vi "Add New Enum Node.vi"(7 "Enum Members":cluster{"Name":string, "Documentation":string}[](array[cluster]), 9 "Type Name":string, 10 "CodeDocumentation":string, 11 "Doc Ref":refnum<k20>) -> (1 "Updated Node Ref":refnum<k20>)   [LabVIEW 2025]
uses:
  <resource>/objmgr/DOMUserDefRef.rc
  Shared/Types/NodeFilteringOptions.ctl
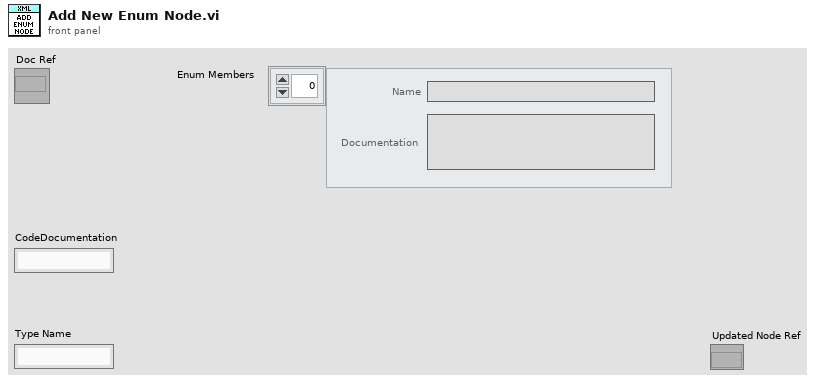
[diagram p1: front panel]
types:
  T1 = typedef "NodeFilteringOptions.ctl" = enum16{"GetCustomDeviceNode", "GetAllChannelNodes", "GetAllSectionNodes", "GetAllWaveformNodes", "GetFirstChannelNode", "GetFirstSectionNode", "GetFirstWaveformNode", "GetSpecificSectionNode", "GetSpecificCustomDeviceNode", "GetSpecificChannelNode", "GetSpecificWaveformNode", "GetMatchedNamedNode", "GetEnumDefinitionsNode", "GetSpecificEnumDefinitionNode", "GetAllEnumDefinitionNodes", "GetDynamicChannelNodes"}
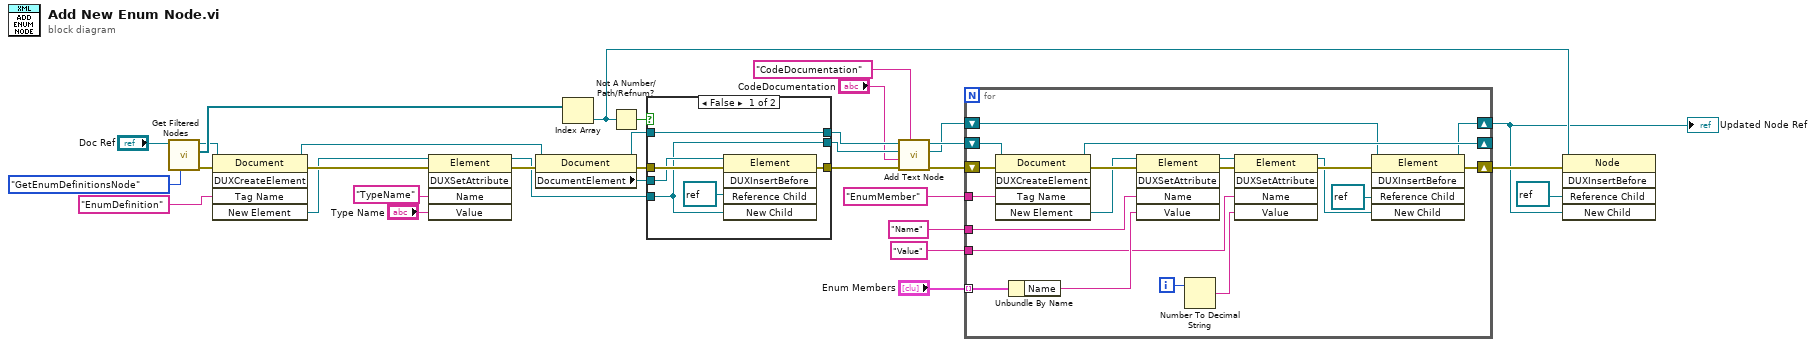
[diagram p0: block diagram]
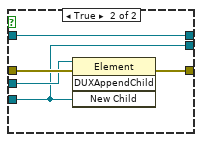
[diagram p2: hidden frame]
diagram:
  n1 = call "Get Filtered Nodes.vi"("Node Filtering"=NodeFilteringOptions."GetEnumDefinitionsNode" ("NodeFiltering"), "Document in"="Doc Ref") -> ("error out"=w22:errorcluster, "Filtered Nodes"=w21:refnum<k20>[], "Document out"=w20:refnum<k20>)  [unwired: 5 in, 2 out]
  n2 = invoke class="Document" method="DUXCreateElement"(reference=w20, error in=w22, "Tag Name"="EnumDefinition") -> (reference out=w24:refnum<k20>, error out=w33:errorcluster, "New Element"=w27:refnum<k20>)  [unwired: 2 in, 2 out]
  n3 = invoke class="Element" method="DUXSetAttribute"(reference=w27, error in=w33, "Name"="TypeName", "Value"="Type Name") -> (reference out=w26:refnum<k20>, error out=w30:errorcluster)  [unwired: 1 in, 3 out]
  n4 = property class="Document"(reference=w24, error in=w30) -> (reference out=w23:refnum<k20>, error out=w25:errorcluster, "DocumentElement"=w29:refnum<k20>)
  n5 = Index Array(array=w21) -> (element=w3:refnum<k20>)  [unwired: 1 in]
  n6 = Not A Number/Path/Refnum?(number/path/refnum=w3) -> (NaN/Path/Refnum?=w28:bool)
  n7 = case shown="False" w28 {
    tunnel: w25 -> [w39 w44]
    tunnel: [w37 w41] -> w17
    tunnel: w26 -> [w35 w40]
    tunnel: w29 -> [w38 w43]
    tunnel: w23 -> [w36 w42]
    tunnel: [w36 w42] -> w15
    tunnel: [w35 w40] -> w16
    frame False {
      n8 = invoke class="Element" method="DUXInsertBefore"(reference=w38, error in=w39, "Reference Child"=refnum<k20> refnum, "New Child"=w35) -> (error out=w37:errorcluster)  [unwired: 1 in, 4 out]
    }
    frame True {
      n9 = invoke class="Element" method="DUXAppendChild"(reference=w43, error in=w44, "New Child"=w40) -> (error out=w41:errorcluster)  [unwired: 1 in, 3 out]
    }
  }
  n10 = call "Add Text Node.vi"("Tag Name"="CodeDocumentation" ("Name"), "error in"=w17, "Tag Data"="CodeDocumentation", "Element in"=w16, "Document in"=w15) -> ("error out"=w12:errorcluster, "Element out"=w6:refnum<k20>, "Document out"=w11:refnum<k20>)  [unwired: 4 in]
  n11 = for {
    shift-right: [w51] -> _
    shift-left: w11 -> [w64]
    tunnel: "EnumMember" ("Tag Name") -> [w62]
    tunnel: "Name" ("Tag Name") -> [w59]
    tunnel: "Enum Members" -> [w58] mode=indexing
    tunnel: "Value" ("Tag Name") -> [w54]
    shift-right: [w46] -> w1
    shift-left: w6 -> [w49]
    shift-right: [w45] -> w4
    shift-left: w12 -> [w63]
    i -> [w53]
    n12 = invoke class="Document" method="DUXCreateElement"(reference=w64, error in=w63, "Tag Name"=w62) -> (reference out=w51:refnum<k20>, error out=w61:errorcluster, "New Element"=w60:refnum<k20>)  [unwired: 2 in, 2 out]
    n13 = Unbundle By Name(w58) -> ("Name"=w57:string)
    n14 = invoke class="Element" method="DUXSetAttribute"(reference=w60, error in=w61, "Name"=w59, "Value"=w57) -> (reference out=w55:refnum<k20>, error out=w56:errorcluster)  [unwired: 1 in, 3 out]
    n15 = Number To Decimal String(number=w53) -> (decimal integer string=w52:string)  [unwired: 1 in]
    n16 = invoke class="Element" method="DUXSetAttribute"(reference=w55, error in=w56, "Name"=w54, "Value"=w52) -> (reference out=w48:refnum<k20>, error out=w50:errorcluster)  [unwired: 1 in, 3 out]
    n17 = invoke class="Element" method="DUXInsertBefore"(reference=w49, error in=w50, "Reference Child"=refnum<k20> refnum, "New Child"=w48) -> (reference out=w46:refnum<k20>, error out=w45:errorcluster)  [unwired: 1 in, 3 out]
  }
  "Updated Node Ref" <- w1
  n18 = invoke class="Node" method="DUXInsertBefore"(reference=w3, error in=w4, "Reference Child"=refnum<k20> refnum, "New Child"=w1) -> ()  [unwired: 1 in, 5 out]
